vi "Run Test Method.vi"(8 "error in (no error)":errorcluster, 11 "LUnit Test Case V2 in":refnum<class "LUnit Test Case V2.lvclass">) -> (0 "error out":errorcluster, 1 "Execution Time":dbl, 3 "LUnit Test Case V2 out":refnum<class "LUnit Test Case V2.lvclass">)   [LabVIEW 2020, in "LUnit Test Case V2.lvclass"]
uses:
  LUnit Test Case V2.lvclass
  LUnit Test Case V2.lvclass/LUnit Test Case V2.ctl
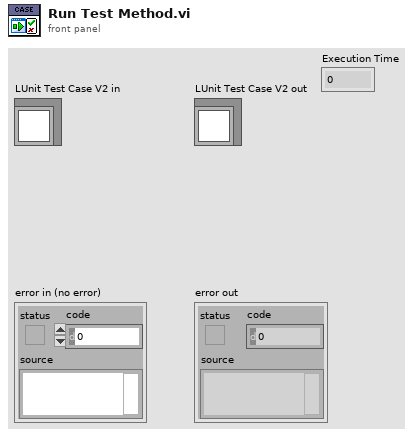
[diagram p1: front panel]
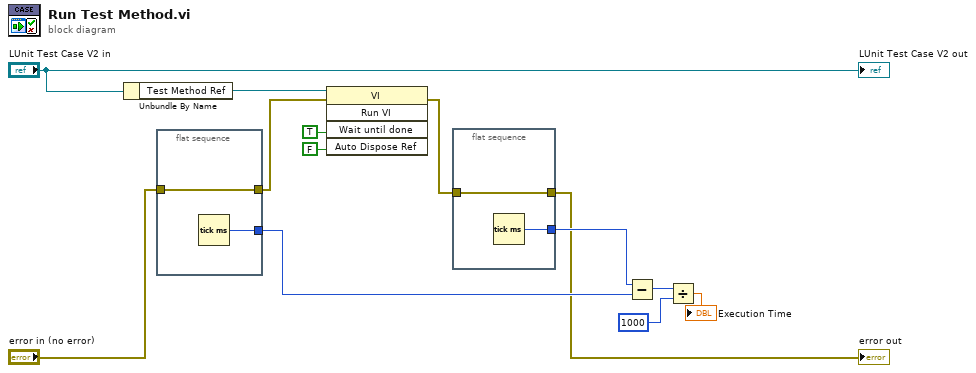
[diagram p0: block diagram]
diagram:
  n1 = Unbundle By Name("LUnit Test Case V2 in") -> ("Test Method Ref"=w2:refnum<vi>)
  n2 = flat-sequence {
    tunnel: "error in (no error)" -> [w15]
    tunnel: [w15] -> w11
    tunnel: [w14] -> w8
    frame #0 {
      n3 = Tick Count (ms)() -> (millisecond timer value=w14:u32)
    }
  }
  n4 = invoke class="VI" method="Run VI"(reference=w2, error in=w11, "Wait until done"=TRUE ("Wait Until Done"), "Auto Dispose Ref"=FALSE ("Auto Dispose Reference")) -> (error out=w10:errorcluster)  [unwired: 1 in, 4 out]
  n5 = flat-sequence {
    tunnel: w10 -> [w17]
    tunnel: [w17] -> w4
    tunnel: [w16] -> w9
    frame #0 {
      n6 = Tick Count (ms)() -> (millisecond timer value=w16:u32)
    }
  }
  n7 = Subtract(x=w9, y=w8) -> (x-y=w7:u32)
  n8 = Divide(x=w7, y=u32 1000) -> (x/y=→"Execution Time":dbl)
  "error out" <- w4
  "LUnit Test Case V2 out" <- "LUnit Test Case V2 in"
